vi "Frequency Modulator.vi"(10 "Waveform In":waveform(dbl), 11 "Carrier Frequency":dbl) -> (2 "Modulated signal":waveform(dbl)(graph), 3 "Radio Spectrum":cluster{"f0":dbl, "df":dbl, "magnitude":dbl[]}(graph))   [LabVIEW 2014, in "Aquisicao de Dados.lvlib"]
uses:
  Aquisicao de Dados.lvlib
  <vilib>/express/express analysis/Spectral/Block/exnSpectralBlock spectral measurements peak poly.vi
  <vilib>/express/express analysis/Spectral/Block/exnSpectralBlock spectral measurements peak WFM.vi
  <vilib>/express/express analysis/Spectral/XNode/ExpressSpectralMeasurementsBlockNode.xnode
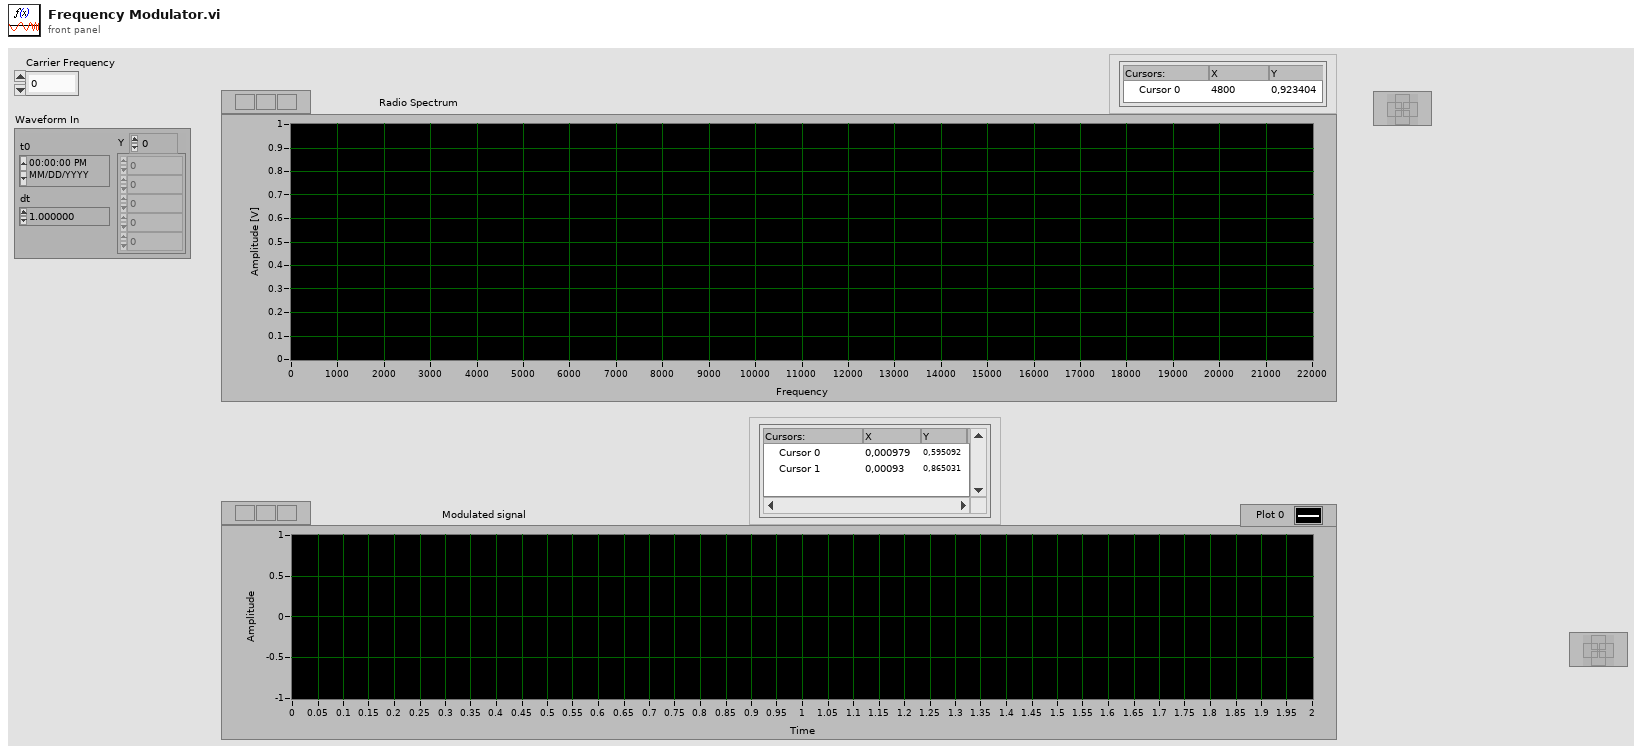
[diagram p1: front panel]
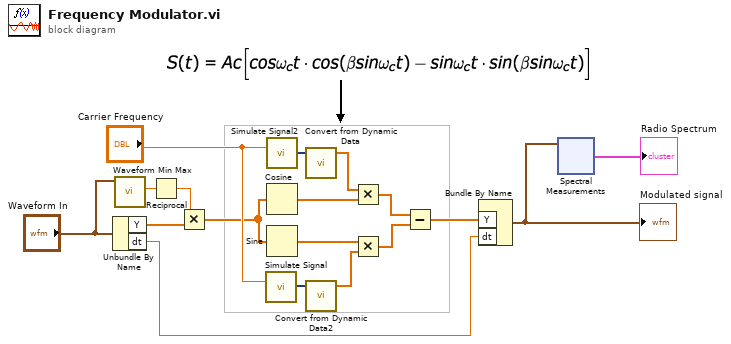
[diagram p0: block diagram]
diagram:
  n1 = Unbundle By Name("Waveform In") -> ("Y"=w10:dbl[], "dt"=w6:dbl)
  n2 = call <vilib>:"Waveform Min Max.vi"("waveform in"="Waveform In") -> ("Y max"=w7:dbl)  [unwired: 5 in, 5 out]
  n3 = Reciprocal(x=w7) -> (1/x=w9:dbl)
  n4 = Multiply(x=w9, y=w10) -> (x*y=w11:dbl[])
  n5 = call "Simulate Signal"("Frequency"="Carrier Frequency") -> ("Sine"=w16:dynamicdata)  [unwired: 13 in, 1 out]
  n6 = call "Simulate Signal2"("Frequency"="Carrier Frequency") -> ("Sine"=w13:dynamicdata)  [unwired: 13 in, 1 out]
  n7 = Cosine(x=w11) -> (cos(x)=w2:dbl[])
  n8 = Sine(x=w11) -> (sin(x)=w3:dbl[])
  n9 = call "Convert from Dynamic Data"("Dynamic Data Type"=w13) -> ("Array"=w14:dbl[])  [unwired: 3 in]
  n10 = call "Convert from Dynamic Data2"("Dynamic Data Type"=w16) -> ("Array"=w15:dbl[])  [unwired: 3 in]
  n11 = Multiply(x=w14, y=w2) -> (x*y=w4:dbl[])
  n12 = Multiply(x=w3, y=w15) -> (x*y=w5:dbl[])
  n13 = Subtract(x=w4, y=w5) -> (x-y=w8:dbl[])
  n14 = Bundle By Name("Y"=w8, "dt"=w6) -> (w1:waveform(dbl))  [unwired: 1 in]
  "Modulated signal" <- w1
  n15 = xnode "Spectral\nMeasurements"("Signals"=w1) -> ("FFT - (Peak)"=→"Radio Spectrum":cluster{"f0":dbl, "df":dbl, "magnitude":dbl[]})  [unwired: 1 in, 2 out]
